vi "View A-Scan_Tianyi.vi"(10 "A-Scan Processed":sgl[](graph), 11 "A-Scan (Raw)":u16[](graph)) -> ()   [LabVIEW 2015]
uses:
  <vilib>/Analysis/NI_AALPro.lvlib
panel:
  out "A-Scan (Raw) 2":sgl[](graph)
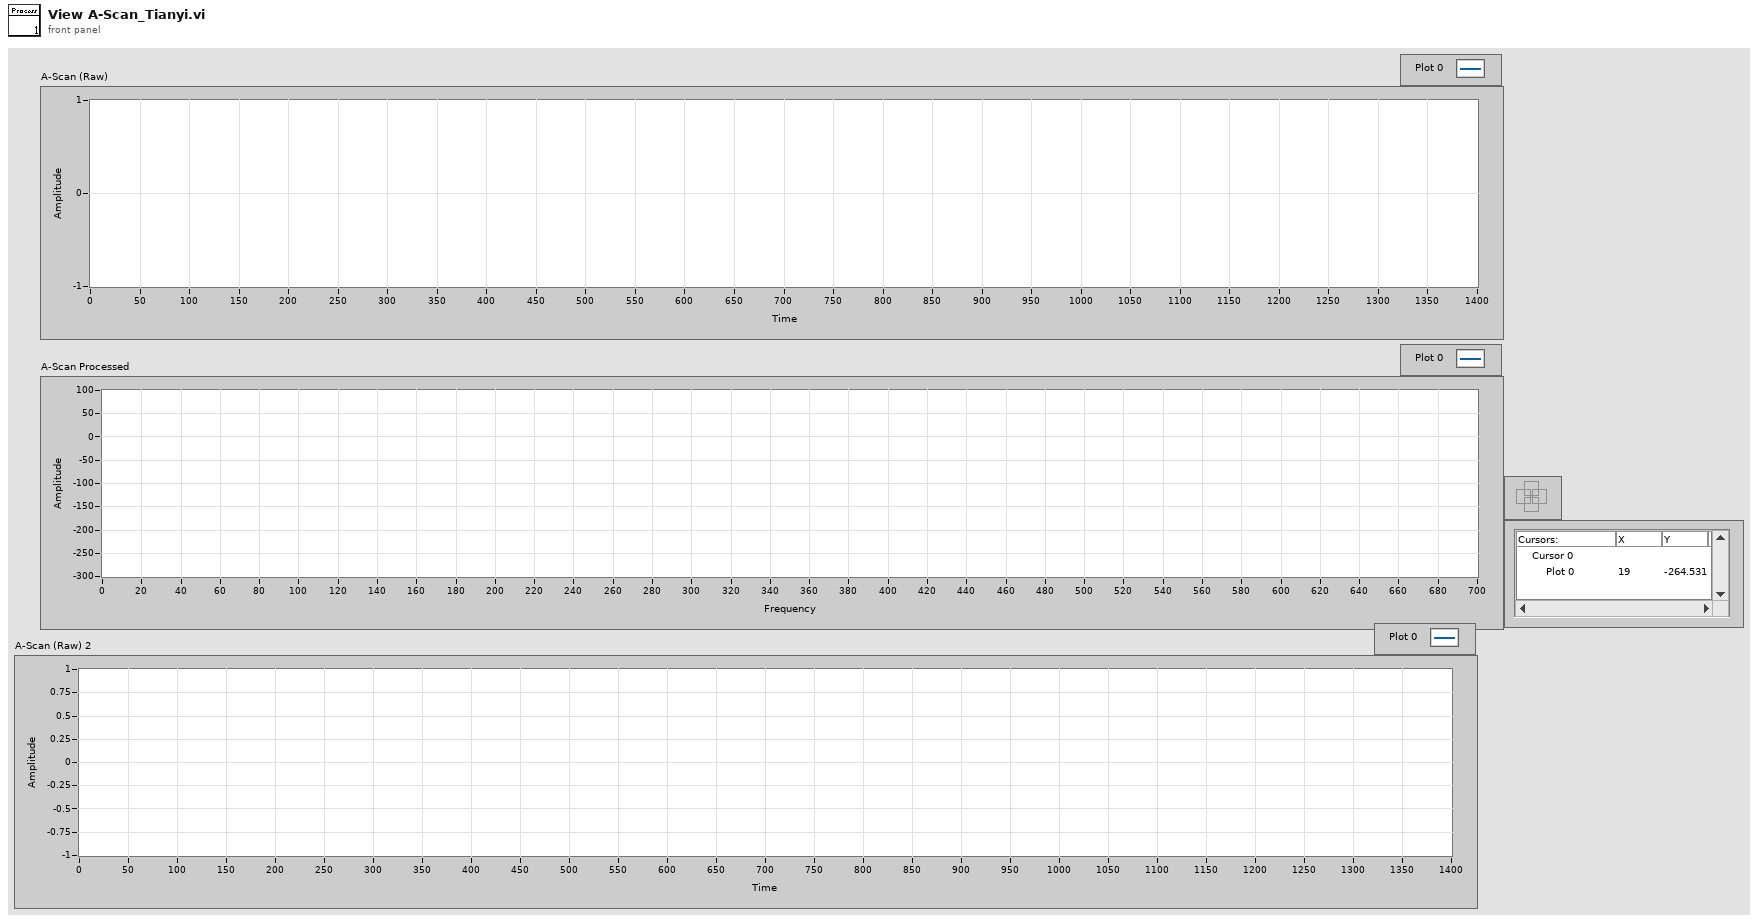
[diagram p1: front panel]
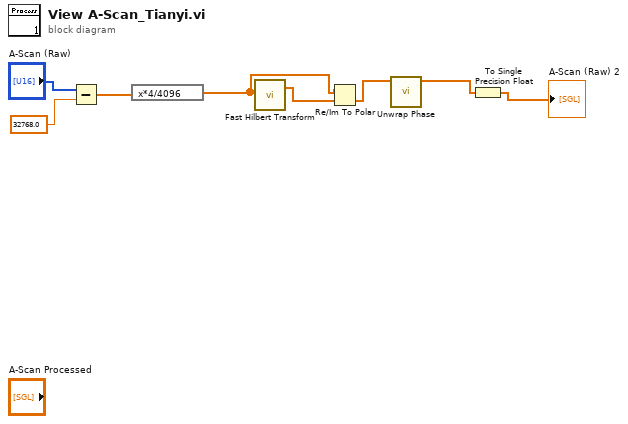
[diagram p0: block diagram]
diagram:
  n1 = Subtract(x="A-Scan (Raw)", y=32768.0) -> (x-y=w6:dbl[])
  n2 = expression code="x*4/4096"(w6) -> (w4:dbl[])
  n3 = call <vilib>:"Fast Hilbert Transform.vi"("X"=w4) -> ("Hilbert{X}"=w5:dbl[])  [unwired: 1 out]
  n4 = Re/Im To Polar(2:w5, 3:w4) -> (0:w3:dbl[])  [unwired: 1 out]
  n5 = call <vilib>:"Unwrap Phase.vi"("Phase"=w3) -> ("Unwrapped Phase"=w1:dbl[])  [unwired: 9 in, 1 out]
  n6 = To Single Precision Float(number=w1) -> (single precision float=→"A-Scan (Raw) 2":sgl[])
